vi "Recenter Panel Bounds.vi"(10 "New Center Coords":T2={"Horizontal"=470, "Vertical"=200}, 11 "Front Panel Window:Panel Bounds in":T1={"Left"=429, "Top"=170, "Right"=540, "Bottom"=313}) -> (3 "Front Panel Window:Panel Bounds out":T1={"Left"=415, "Top"=129, "Right"=526, "Bottom"=129})   [LabVIEW 2018]
uses:
  <vilib>/Utility/miscctls.llb/LVPoint32TypeDef.ctl
  <vilib>/Utility/miscctls.llb/LVRectTypeDef.ctl
panel:
  out "Y change":i32=-41
  out "X change":i32=-14
  out "old center Y":i16=241
  out "old center X":i16=484
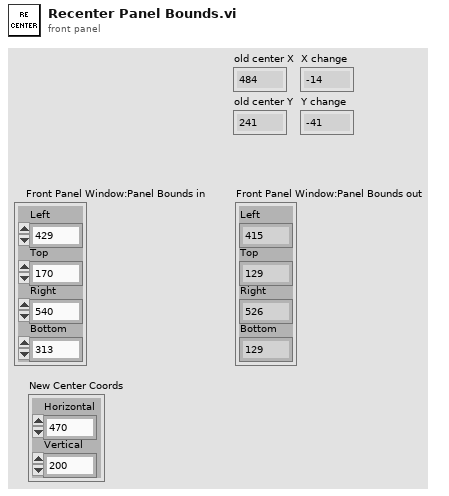
[diagram p1: front panel]
types:
  T1 = typedef "LVRectTypeDef.ctl" = cluster{"Left":i16, "Top":i16, "Right":i16, "Bottom":i16}
  T2 = typedef "LVPoint32TypeDef.ctl" = cluster{"Horizontal":i32, "Vertical":i32}
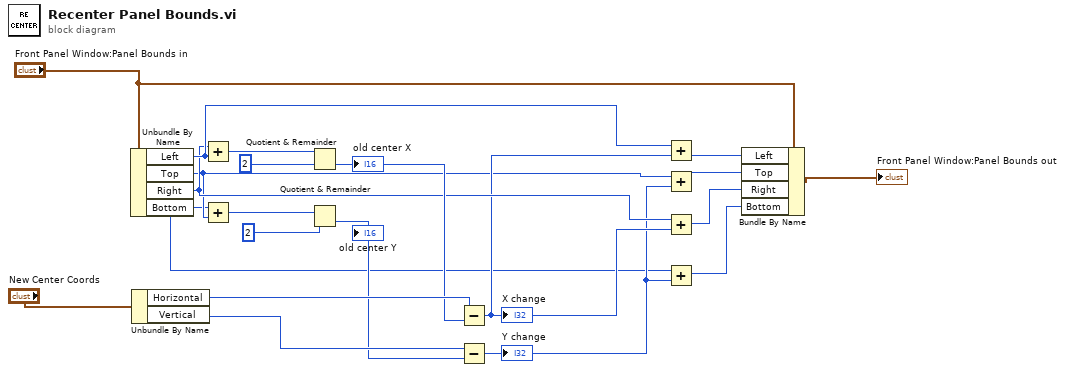
[diagram p0: block diagram]
diagram:
  n1 = Unbundle By Name("Front Panel Window:Panel Bounds in") -> ("Left"=w12:i16, "Top"=w8:i16, "Right"=w11:i16, "Bottom"=w1:i16)
  n2 = Unbundle By Name("New Center Coords") -> ("Horizontal"=w16:i32, "Vertical"=w14:i32)
  n3 = Add(x=w11, y=w12) -> (x+y=w21:i16)
  n4 = Add(x=w1, y=w8) -> (x+y=w19:i16)
  n5 = Quotient & Remainder(x=w21, y=i16 2) -> (floor(x/y)=w15:i16)  [unwired: 1 out]
  "old center X" <- w15
  n6 = Quotient & Remainder(x=w19, y=i16 2) -> (floor(x/y)=w13:i16)  [unwired: 1 out]
  "old center Y" <- w13
  n7 = Subtract(x=w16, y=w15) -> (x-y=w10:i32)
  "X change" <- w10
  n8 = Subtract(x=w14, y=w13) -> (x-y=w9:i32)
  "Y change" <- w9
  n9 = Add(x=w12, y=w10) -> (x+y=w6:i32)
  n10 = Add(x=w8, y=w9) -> (x+y=w5:i32)
  n11 = Add(x=w11, y=w10) -> (x+y=w4:i32)
  n12 = Add(x=w1, y=w9) -> (x+y=w3:i32)
  n13 = Bundle By Name(cluster="Front Panel Window:Panel Bounds in", "Left"=w6, "Top"=w5, "Right"=w4, "Bottom"=w3) -> (→"Front Panel Window:Panel Bounds out":T1)
